vi "DoubleLongProbe.vi"() -> ()   [LabVIEW 2010]
panel:
  out "DoubleLong":dbl
  in  "Probe":dbl
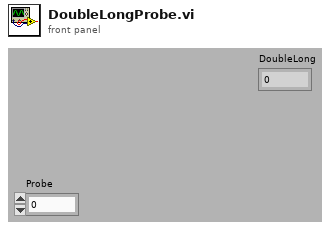
[diagram p1: front panel]
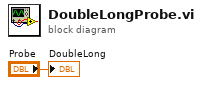
[diagram p0: block diagram]
diagram:
  "DoubleLong" <- "Probe"
